vi "Init Vecto.vi"(8 "error in (no error)":errorcluster, 11 "Volatus Core in":refnum<class "Volatus Core.lvclass">) -> (0 "error out":errorcluster, 3 "Volatus Core out":refnum<class "Volatus Core.lvclass">)   [LabVIEW 2020, in "Volatus.lvlib" / "Volatus Core.lvclass"]
uses:
  Volatus Core.lvclass
  C:/dev/lv20CE/relink/lv-volatus/Volatus/Module/Module.lvclass
  lv-vecto/Vecto/Event Level.ctl
  lv-vecto/Vecto/Init Implementations.ctl
  lv-vecto/Vecto/EventLogHandler/EventLogHandler.lvclass
  Volatus Core.lvclass/Volatus Core.ctl
  Module/Module.lvclass/Module.ctl
  VectoEventBridge/VectoEventBridge.lvclass
  C:/dev/lv20CE/relink/lv-vecto/Vecto/EventLogHandler/EventLogHandler.lvclass
  Module/Module.lvclass
  lv-vecto/Vecto/Vecto/Vecto.lvclass
  lv-vecto/Vecto/Vecto.lvlib
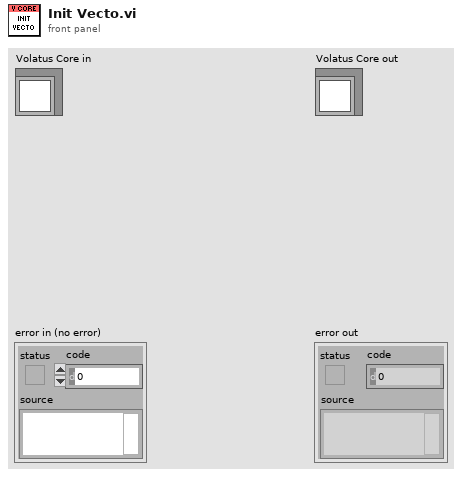
[diagram p1: front panel]
types:
  T1 = typedef "Vecto.lvlib/Init Implementations.ctl" = cluster{"EventLogger":refnum<class "EventLogHandler.lvclass">}
  T2 = typedef "Vecto.lvlib/Event Level.ctl" = enum16{"Debug", "Info", "Warning", "Error"}
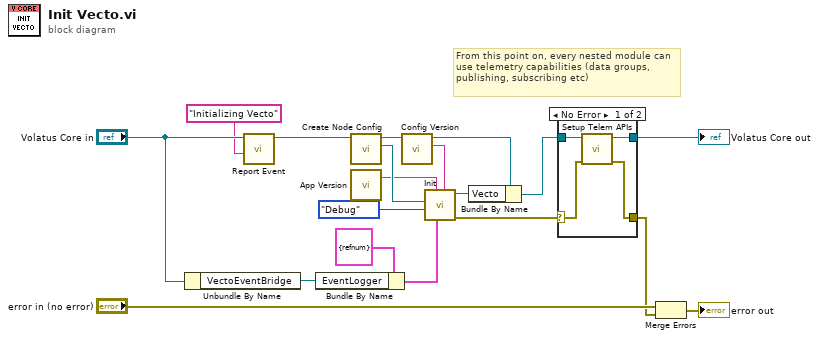
[diagram p0: block diagram]
diagram:
  # "From this point on, every nested module can use telemetry capabilities (data groups, publishing, subscribing etc)"
  n1 = Unbundle By Name("Volatus Core in") -> ("VectoEventBridge"=w13:refnum<class "VectoEventBridge.lvclass">)
  n2 = call "Report Event.vi"("Message"="Initializing Vecto", "Module in"="Volatus Core in") -> ("Module out"=w2:refnum<class "Volatus Core.lvclass">)  [unwired: 8 in, 1 out]
  n3 = Bundle By Name(cluster=T1 {"EventLogger"=refnum} ("Init Implementations"), "EventLogger"=w13) -> (w15:T1)
  n4 = call "Create Node Config.vi"("Volatus Core in"=w2) -> ("Node"=w17:refnum<class "Node Config.lvclass">, "Volatus Core out"=w11:refnum<class "Volatus Core.lvclass">)  [unwired: 8 in, 1 out]
  n5 = call "App Version.vi"() -> ("App Version"=w12:string)  [unwired: 3 in]
  n6 = call "Config Version.vi"("Volatus Core in"=w11) -> ("Config Version"=w10:string, "Volatus Core out"=w9:refnum<class "Volatus Core.lvclass">)  [unwired: 8 in, 1 out]
  n7 = call "Init.vi"("Config Version"=w10, "Init Implementations"=w15, "App Version"=w12, "Minimum Event Level (Info)"=Event_Level."Debug", "Node"=w17) -> ("error out"=w5:errorcluster, "Vecto out"=w7:refnum<class "Vecto.lvclass">)  [unwired: 5 in]
  n8 = Bundle By Name(cluster=w9, "Vecto"=w7) -> (w8:refnum<class "Volatus Core.lvclass">)
  n9 = case shown="No Error" w5 {
    selector: w5 -> [w21 w24]
    tunnel: w8 -> [w23 w25]
    tunnel: [w22 w25] -> w6
    tunnel: [w20 w24] -> w3
    frame No Error {
      n10 = call "Setup Telem APIs.vi"("error in (no error)"=w21, "Volatus Core in"=w23) -> ("error out"=w20:errorcluster, "Volatus Core out"=w22:refnum<class "Volatus Core.lvclass">)  [unwired: 8 in]
    }
    frame Error {
    }
  }
  "Volatus Core out" <- w6
  n11 = Merge Errors("error in (no error)", w3) -> (→"error out":errorcluster)
